vi "GET_RESULT.vi"(7 "LabVIEW Web Service Request":refnum<class "Web Request.lvclass">, 11 "DEVICE_SN":string) -> (3 "Response":T1)   [LabVIEW 2015]
uses:
  <vilib>/wsapi/Web Request.lvclass
  Share Data/uPower_kit.ctl
panel:
  # "Use the Web Service Request input terminal to call the VIs on the Web Services palette. Do not remove it from the connector pane unless you don't need access to the palette."
  # "Each additional control wired to the connector pane will be available as an input in the URL. To include an indicator in terminal-mode output (the default setting), it must also be wired to the connector pane."
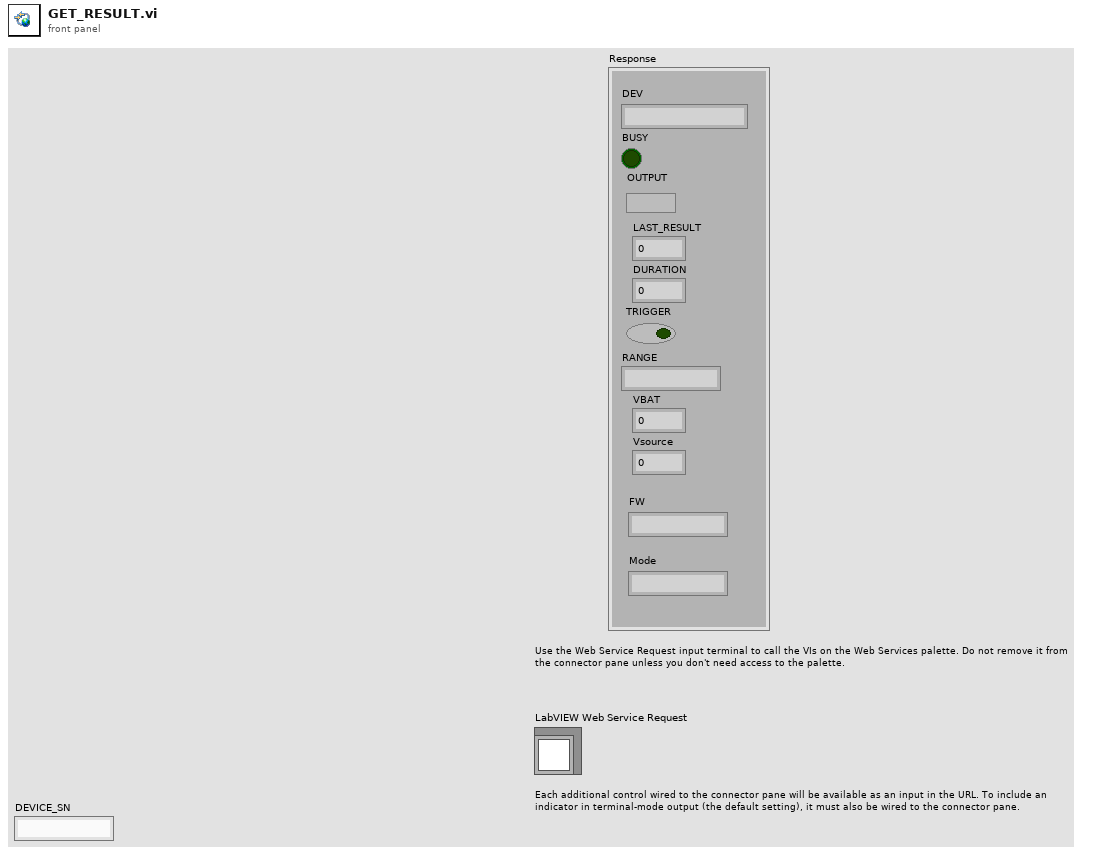
[diagram p1: front panel]
types:
  T1 = typedef "uPower_kit.ctl" = cluster{"DEV":string, "BUSY":bool, "VBAT":dbl, "OUTPUT":bool, "LAST_RESULT":dbl, "DURATION":u16, "TRIGGER":bool, "RANGE":string, "Vsource":dbl, "FW":string, "Mode":string}
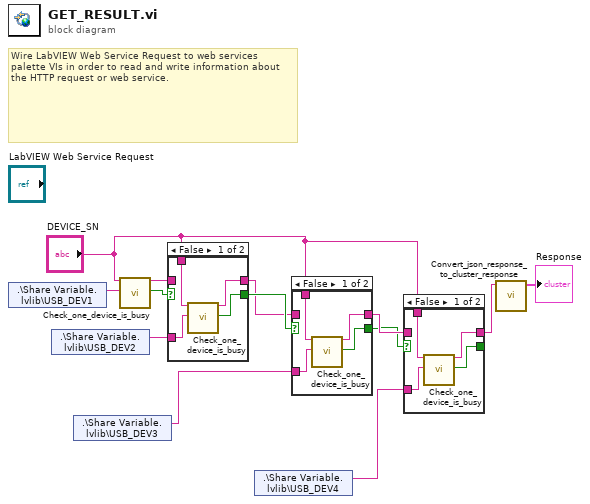
[diagram p0: block diagram]
diagram:
  # "Wire LabVIEW Web Service Request to web services palette VIs in order to read and write information about the HTTP request or web service."
  n1 = shared-variable ".\\Share Variable.lvlib\\USB_DEV1"() -> (w10:string)  [unwired: 1 in, 1 out]
  n2 = shared-variable ".\\Share Variable.lvlib\\USB_DEV2"() -> (w12:string)  [unwired: 1 in, 1 out]
  n3 = shared-variable ".\\Share Variable.lvlib\\USB_DEV3"() -> (w7:string)  [unwired: 1 in, 1 out]
  n4 = call "Check_one_device_is_busy.vi"("DEVICE_SN"="DEVICE_SN", "USB_DEV_json"=w10) -> ("USB_DEV_Json"=w13:string, "Device?"=w11:bool)  [unwired: 16 in]
  n5 = case shown="False" w11 {
    selector: w11 -> [_ w19]
    tunnel: w12 -> [w17 _]
    tunnel: [w16 w19] -> w8
    tunnel: [w15 w18] -> w6
    tunnel: w13 -> [_ w18]
    tunnel: "DEVICE_SN" -> [w14 _]
    frame False {
      n6 = call "Check_one_device_is_busy.vi"("DEVICE_SN"=w14, "USB_DEV_json"=w17) -> ("USB_DEV_Json"=w15:string, "Device?"=w16:bool)  [unwired: 16 in]
    }
    frame True {
    }
  }
  n7 = shared-variable ".\\Share Variable.lvlib\\USB_DEV4"() -> (w5:string)  [unwired: 1 in, 1 out]
  n8 = case shown="False" w8 {
    selector: w8 -> [_ w25]
    tunnel: w7 -> [w23 _]
    tunnel: [w22 w25] -> w3
    tunnel: [w21 w24] -> w4
    tunnel: w6 -> [_ w24]
    tunnel: "DEVICE_SN" -> [w20 _]
    frame False {
      n9 = call "Check_one_device_is_busy.vi"("DEVICE_SN"=w20, "USB_DEV_json"=w23) -> ("USB_DEV_Json"=w21:string, "Device?"=w22:bool)  [unwired: 16 in]
    }
    frame True {
    }
  }
  n10 = case shown="False" w3 {
    selector: w3 -> [_ w31]
    tunnel: w5 -> [w29 _]
    tunnel: [w28 w31] -> _
    tunnel: [w27 w30] -> w2
    tunnel: w4 -> [_ w30]
    tunnel: "DEVICE_SN" -> [w26 _]
    frame False {
      n11 = call "Check_one_device_is_busy.vi"("DEVICE_SN"=w26, "USB_DEV_json"=w29) -> ("USB_DEV_Json"=w27:string, "Device?"=w28:bool)  [unwired: 16 in]
    }
    frame True {
    }
  }
  n12 = call "Convert_json_response_to_cluster_response.vi"("Json_Response_in"=w2) -> ("Response"=→"Response":T1)  [unwired: 10 in]
